vi "Fetch Multiple Points.vi"(8 "error in (no error)":errorcluster, 9 "Timeout (10000 ms)":i32=10000 format="%#.6g", 11 "VISA resource name":refnum<visa-resource-name>) -> (0 "error out":errorcluster, 2 "Measurements":dbl[](array[numeric]), 3 "VISA resource name out":refnum<visa-resource-name>)   [LabVIEW 2020, in "Agilent 3446X Series.lvlib"]
doc: "This low-level VI returns an array of values from a previously initiated measurement. The number of measurements the DMM takes is determined by the values you specify for the <B>Trigger Count</B> control and <B>Sample Count</B> control of the Configure Multipoint VI.\n\n<B>Note:</B> Use this VI only with other low-level VIs. The high-level VIs automatically incorporate this functionality. This VI does not check the instrument status. If you want to check the instrument status, call the Error Query VI at the conclusion of the sequence."
uses:
  Agilent 3446X Series.lvlib
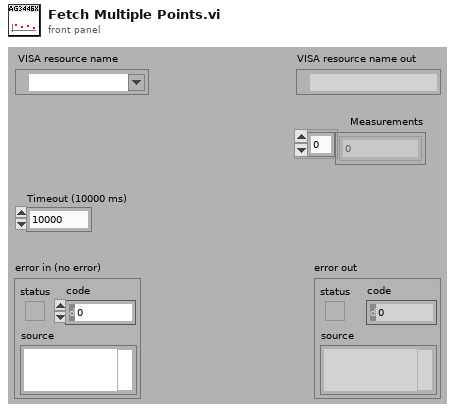
[diagram p1: front panel]
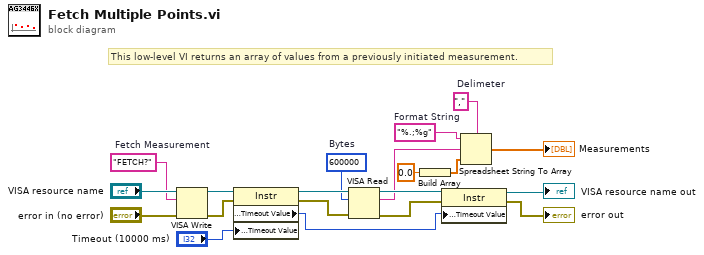
[diagram p0: block diagram]
diagram:
  w16 = ","  # Delimeter
  w17 = "%.;%g"  # Format String
  w18 = "FETCH?"  # Fetch Measurement
  w1 = u32 600000  # Bytes
  # "This low-level VI returns an array of values from a previously initiated measurement."
  n1 = VISA Write(VISA resource name="VISA resource name", write buffer=w18, error in (no error)="error in (no error)") -> (VISA resource name out=w12:refnum<visa-resource-name>, error out=w11:errorcluster)  [unwired: 1 out]
  n2 = property class="Instr"(reference=w12, error in=w11, "General Settings:Timeout Value"="Timeout (10000 ms)") -> (reference out=w10:refnum<visa-resource-name>, error out=w9:errorcluster, "General Settings:Timeout Value"=w5:u32)
  n3 = VISA Read(VISA resource name=w10, byte count=w1, error in (no error)=w9) -> (VISA resource name out=w7:refnum<visa-resource-name>, read buffer=w2:string, error out=w6:errorcluster)  [unwired: 1 out]
  n4 = Build Array(0.0) -> (w14:dbl[])
  n5 = property class="Instr"(reference=w7, error in=w6, "General Settings:Timeout Value"=w5) -> (reference out=→"VISA resource name out":refnum<visa-resource-name>, error out=→"error out":errorcluster)
  n6 = Spreadsheet String To Array(delimiter (Tab)=w16, format string=w17, spreadsheet string=w2, array type (2D Dbl)=w14) -> (array=→"Measurements":dbl[])
